vi "Parallel RGB to Grayscale.vi"(7 "Depth?":bool, 8 "Pixel Queue Float":refnum<queue>, 9 "Pixel Queue":refnum<queue>, 10 "Coordinate":T1, 11 "Image Pixels (U32)":u32[][](array[numeric])) -> ()   [LabVIEW 2018]
uses:
  Pixel Data STYP.ctl
  Coordinate STYP.ctl
  Floating Pixel Data STYP.ctl
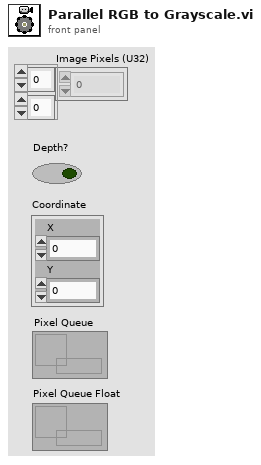
[diagram p1: front panel]
types:
  T1 = typedef "Coordinate STYP.ctl" = cluster{"X":i32, "Y":i32}
  T2 = typedef "Pixel Data STYP.ctl" = cluster{"Value":u8, "Coordinate":T1}
  T3 = typedef "Floating Pixel Data STYP.ctl" = cluster{"Value":dbl, "Coordinate":T1}
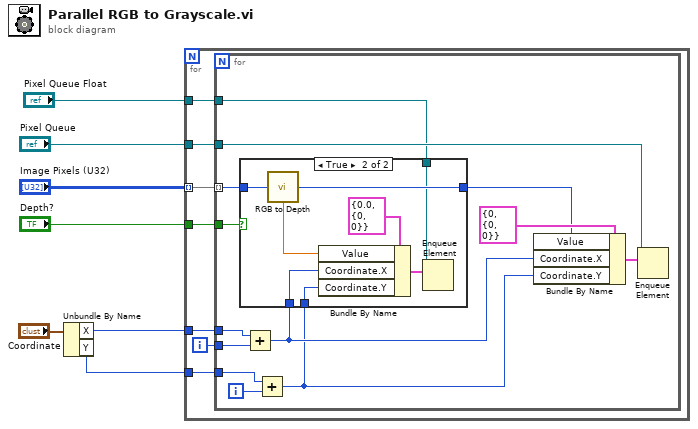
[diagram p0: block diagram]
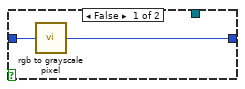
[diagram p2: hidden frame]
diagram:
  n1 = Unbundle By Name("Coordinate") -> ("X"=w4:i32, "Y"=w3:i32)
  n2 = for {
    tunnel: "Image Pixels (U32)" -> [w14] mode=indexing
    tunnel: "Pixel Queue" -> [w13]
    tunnel: w4 -> [w11]
    tunnel: w3 -> [w10]
    tunnel: "Depth?" -> [w9]
    tunnel: "Pixel Queue Float" -> [w8]
    i -> [w12]
    n3 = for {
      tunnel: w14 -> [w27] mode=indexing
      tunnel: w13 -> [w23]
      tunnel: w12 -> [w25]
      tunnel: w11 -> [w21]
      tunnel: w10 -> [w20]
      tunnel: w9 -> [w18]
      tunnel: w8 -> [w17]
      i -> [w19]
      n4 = Add(x=w21, y=w25) -> (x+y=w16:i32)
      n5 = Add(x=w20, y=w19) -> (x+y=w15:i32)
      n6 = case shown="True" w18 {
        tunnel: w27 -> [w29 w37]
        tunnel: [w28 w36] -> w24
        tunnel: w17 -> [_ w35]
        tunnel: w16 -> [_ w31]
        tunnel: w15 -> [_ w30]
        frame False {
          n7 = call "rgb to grayscale pixel.vi"("Color (U32)"=w29) -> ("Grayscale (U8)"=w28:u8)  [unwired: 14 in]
        }
        frame True {
          n8 = call "RGB to Depth.vi"("RGB"=w37) -> ("Depth Pixel"=w36:u8, "Depth"=w32:dbl)  [unwired: 13 in]
          n9 = Bundle By Name(cluster=T3 {"Value"=0.0, "Coordinate"={"X"=0, "Y"=0}} ("Data"), "Value"=w32, "Coordinate.X"=w31, "Coordinate.Y"=w30) -> (w34:T3)
          n10 = Enqueue Element(queue=w35, element=w34) -> ()  [unwired: 2 in, 3 out]
        }
      }
      n11 = Bundle By Name(cluster=T2 {"Value"=0, "Coordinate"={"X"=0, "Y"=0}} ("Data"), "Value"=w24, "Coordinate.X"=w16, "Coordinate.Y"=w15) -> (w22:T2)
      n12 = Enqueue Element(queue=w23, element=w22) -> ()  [unwired: 2 in, 3 out]
    }
  }
